vi "Read Transmission Data Unit.vi"(8 "error in":errorcluster, 11 "Modbus instance in":refnum<class "Modbus Master.lvclass">) -> (0 "error out":errorcluster, 2 "transmission data unit":refnum<class "Transmission Data Unit.lvclass">, 3 "Modbus instance out":refnum<class "Modbus Master.lvclass">)   [LabVIEW 2021, in "Modbus Master.lvclass"]
doc: "This VI is an accessor for the transmission data unit stored in the Modbus instance. This accessor can be used as a property node. The transmission data unit is used by the device to determine how to pack and unpack data coming from the physical bus."
uses:
  Modbus Master.lvclass
  Modbus Master.lvclass/Modbus Master.ctl
  Network Protocol/Network Master/Network Master.lvclass
  Transmission Data Unit/Transmission Data Unit.lvclass
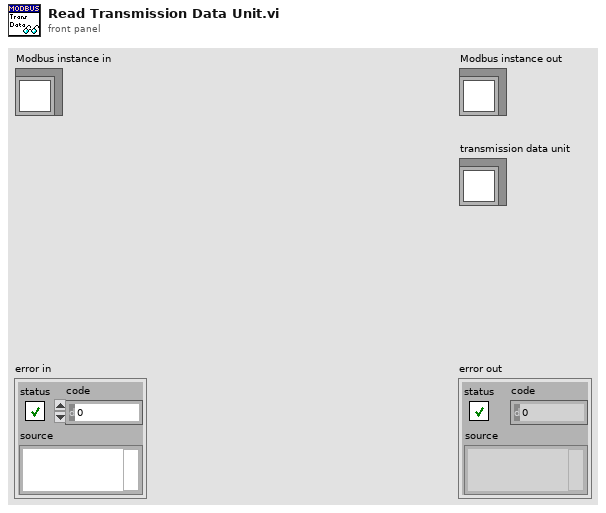
[diagram p1: front panel]
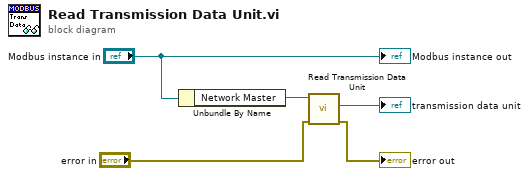
[diagram p0: block diagram]
diagram:
  n1 = Unbundle By Name("Modbus instance in") -> ("Network Master"=w4:refnum<class "Network Master.lvclass">)
  n2 = call "Read Transmission Data Unit.vi"("error in (no error)"="error in", "Network Master in"=w4) -> ("error out"=→"error out":errorcluster, "Transmission Data Unit"=→"transmission data unit":refnum<class "Transmission Data Unit.lvclass">)  [unwired: 7 in, 1 out]
  "Modbus instance out" <- "Modbus instance in"
